vi "Get Acquisition Timings.vi"(9 "kinetic":sgl, 10 "accumulate":sgl, 11 "exposure":sgl) -> (1 "kinetic out":sgl, 2 "accumulate out":sgl, 3 "exposure out":sgl, 5 "function return":u32)   [LabVIEW 2018, in "AndorSDK.lvlib"]
doc: "EXPNETTYPE unsigned int WINAPI GetAcquisitionTimings(float * exposure, float * accumulate, float * kinetic);"
uses:
  AndorSDK.lvlib
  ATMCD32D.dll
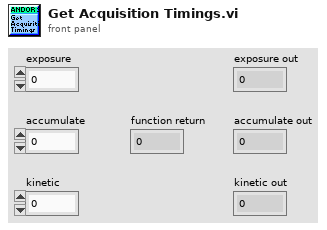
[diagram p1: front panel]
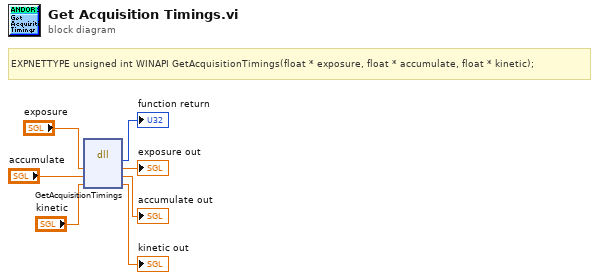
[diagram p0: block diagram]
diagram:
  # "EXPNETTYPE unsigned int WINAPI GetAcquisitionTimings(float * exposure, float * accumulate, float * kinetic);"
  n1 = dll-call lib="PTH2babs E\nPersönliches02 - Arbeit03-HiwijobsLabviewCodelibANDOR\tAndor SDK\nATMCD32D.*" fn="GetAcquisitionTimings"("exposure"="exposure", "accumulate"="accumulate", "kinetic"="kinetic") -> (→"function return":u32, "exposure"=→"exposure out":sgl, "accumulate"=→"accumulate out":sgl, "kinetic"=→"kinetic out":sgl)  [unwired: 3 in, 2 out]
